vi "Unix Epoch to Timestamp.vi"(10 "error in (no error)":errorcluster, 11 "Unix Epoch Seconds":dbl format="%#.6f") -> (2 "error out":errorcluster, 3 "Time Stamp":timestamp)   [LabVIEW 2020, in "JWT.lvlib"]
uses:
  JWT.lvlib
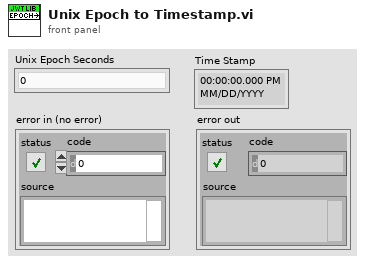
[diagram p1: front panel]
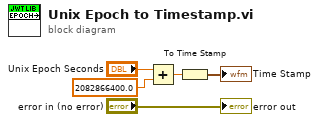
[diagram p0: block diagram]
diagram:
  n1 = Add(x="Unix Epoch Seconds", y=2082866400.0 ("double precision float")) -> (x+y=w2:dbl)
  n2 = To Time Stamp(1:w2) -> (0:→"Time Stamp":timestamp)
  "error out" <- "error in (no error)"
